vi "VNA_Set_Selected_Measurement.vi"(2 "error in (no error)":errorcluster, 3 "VISA in":refnum<visa-resource-name>) -> (0 "error out":errorcluster, 1 "VISA out":refnum<visa-resource-name>)   [LabVIEW 2017]
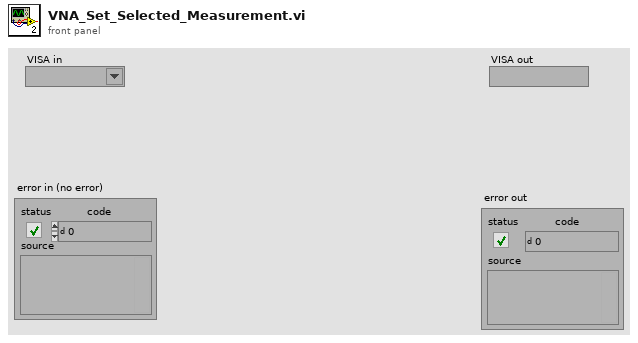
[diagram p1: front panel]
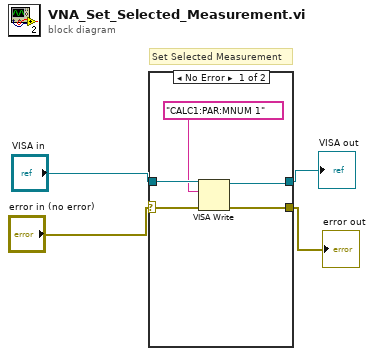
[diagram p0: block diagram]
diagram:
  # "Set Selected Measurement"
  n1 = case shown="No Error" "error in (no error)" {
    selector: "error in (no error)" -> [w9 w11]
    tunnel: [w5 w11] -> w2
    tunnel: "VISA in" -> [w8 w10]
    tunnel: [w6 w10] -> w1
    frame No Error {
      n2 = VISA Write(VISA resource name=w8, write buffer="CALC1:PAR:MNUM 1" ("Cmdline"), error in (no error)=w9) -> (VISA resource name out=w6:refnum<visa-resource-name>, error out=w5:errorcluster)  [unwired: 1 out]
    }
    frame Error {
    }
  }
  "error out" <- w2
  "VISA out" <- w1
